vi "Update Color Table.vi"(8 "error in (no error)":errorcluster, 10 "Color Table":T1={"Occupied Color"={"Value"=0, "Color"=0}, "Free Color"={"Value"=205, "Color"=16777215}, "Unknown Color"={"Value"=254, "Color"=13421772}}, 11 "Map Model in":refnum<class "Map Model.lvclass">) -> (0 "error out":errorcluster, 3 "Map Model out":refnum<class "Map Model.lvclass">)   [LabVIEW 2020, in "Map Model.lvlib" / "Map Model.lvclass"]
uses:
  Map Model.lvclass
  Map Model.lvclass/Map Model.ctl
panel:
  # "NOTICE -- YOU MUST LEAVE THIS NOTICE IN PLACE.\n\nCopyright (c) 2017, LIANG LIU Shawn.Liu.cn@gmail.com\nAll rights reserved.\n\nRedistribution and use in source and binary forms, with or without modification, are permitted provided that the following conditions are met:\n-Redistributions of source code must retain the above copyright notice, this list of conditions and the following disclaimer.\n-Redistributions in binary form must reproduce the above copyright notice, this list of conditions and the following disclaimer in the documentation and/or other materials provided with the distribution.\n-Neither the name of the eLp nor the names of its contributors may be used to endorse or promote products derived from this software without specific prior written permission.\n\nTHIS SOFTWARE IS PROVIDED BY THE COPYRIGHT HOLDERS AND CONTRIBUTORS \"AS IS\" AND ANY EXPRESS OR IMPLIED WARRANTIES, INCLUDING, BUT NOT LIMITED TO, THE IMPLIED WARRANTIES OF MERCHANTABILITY AND FITNESS FOR A PARTICULAR PURPOSE ARE DISCLAIMED. IN NO EVENT SHALL THE COPYRIGHT HOLDER OR CONTRIBUTORS BE LIABLE FOR ANY DIRECT, INDIRECT, INCIDENTAL, SPECIAL, EXEMPLARY, OR CONSEQUENTIAL DAMAGES (INCLUDING, BUT NOT LIMITED TO, PROCUREMENT OF SUBSTITUTE GOODS OR SERVICES; LOSS OF USE, DATA, OR PROFITS; OR BUSINESS INTERRUPTION) HOWEVER CAUSED AND ON ANY THEORY OF LIABILITY, WHETHER IN CONTRACT, STRICT LIABILITY, OR TORT (INCLUDING NEGLIGENCE OR OTHERWISE) ARISING IN ANY WAY OUT OF THE USE OF THIS SOFTWARE, EVEN IF ADVISED OF THE POSSIBILITY OF SUCH DAMAGE."
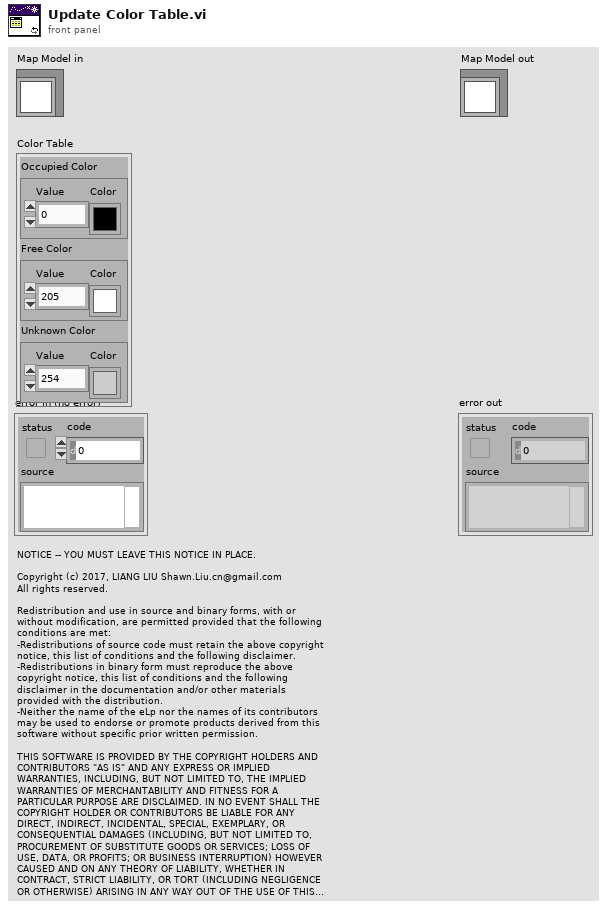
[diagram p1: front panel]
types:
  T1 = cluster{"Occupied Color":cluster{"Value":u8, "Color":u32}, "Free Color":cluster{"Value":u8, "Color":u32}, "Unknown Color":cluster{"Value":u8, "Color":u32}}
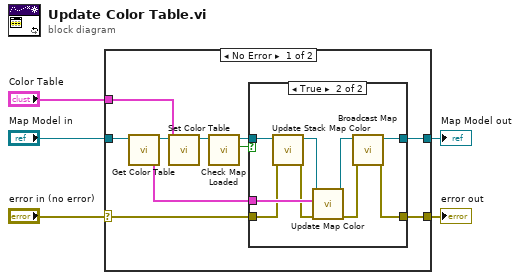
[diagram p0: block diagram]
diagram:
  n1 = case shown="No Error" "error in (no error)" {
    selector: "error in (no error)" -> [w11 w28]
    tunnel: "Map Model in" -> [w15 w27]
    tunnel: [w14 w27] -> w4
    tunnel: "Color Table" -> [w13 _]
    tunnel: [w12 w28] -> w2
    frame No Error {
      n2 = call "Get Color Table.vi"("Map Model in"=w15) -> ("Color Table"=w6:T1, "Map Model out"=w7:refnum<class "Map Model.lvclass">)  [unwired: 9 in]
      n3 = call "Set Color Table.vi"("Color Table"=w13, "Map Model in"=w7) -> ("Map Model out"=w10:refnum<class "Map Model.lvclass">)  [unwired: 9 in]
      n4 = call "Check Map Loaded.vi"("Map Model in"=w10) -> ("Loaded"=w8:bool, "Map Model out"=w9:refnum<class "Map Model.lvclass">)  [unwired: 9 in]
      n5 = case shown="True" w8 {
        tunnel: [w17 w26] -> w14
        tunnel: [w16 w25] -> w12
        tunnel: w9 -> [w17 w24]
        tunnel: w11 -> [w16 w22]
        tunnel: w6 -> [_ w23]
        frame False {
        }
        frame True {
          n6 = call "Update Stack Map Color.vi"("error in (no error)"=w22, "Map Model in"=w24) -> ("error out"=w21:errorcluster, "Map Model out"=w20:refnum<class "Map Model.lvclass">)  [unwired: 8 in]
          n7 = call "Update Map Color.vi"("error in (no error)"=w21, "Old Color Table"=w23, "Map Model in"=w20) -> ("error out"=w18:errorcluster, "Map Model out"=w19:refnum<class "Map Model.lvclass">)  [unwired: 7 in]
          n8 = call "Broadcast Map.vi"("error in (no error)"=w18, "Map Model in"=w19) -> ("error out"=w25:errorcluster, "Map Model out"=w26:refnum<class "Map Model.lvclass">)  [unwired: 8 in]
        }
      }
    }
    frame Error {
    }
  }
  "error out" <- w2
  "Map Model out" <- w4
